vi "Step by Name or ID.vi"(8 "error in (no error)":errorcluster, 10 "Name or ID":string, 11 "Sequence in":refnum<class "Sequence.lvclass">) -> (0 "error out":errorcluster, 2 "Step":refnum<class "Step.lvclass">, 3 "Sequence out":refnum<class "Sequence.lvclass">)   [LabVIEW 2020, in "TSnax.lvlib" / "Sequence.lvclass"]
uses:
  Sequence.lvclass
  Sequence.lvclass/Sequence.ctl
  Step/Step.lvclass
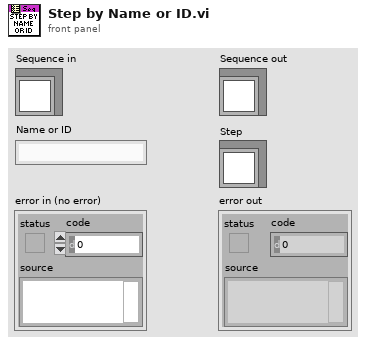
[diagram p1: front panel]
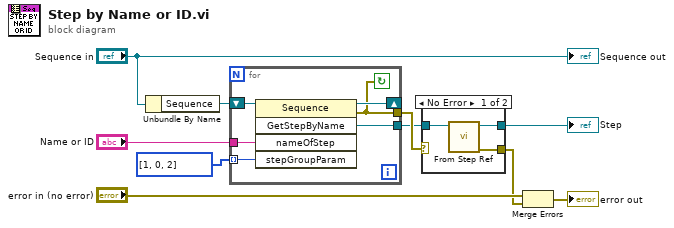
[diagram p0: block diagram]
diagram:
  n1 = Unbundle By Name("Sequence in") -> ("Sequence"=w7:refnum<k7>)
  n2 = for {
    tunnel: "Name or ID" -> [w15]
    tunnel: i32[] [1, 0, 2] -> [w14] mode=indexing
    shift-right: [w13] -> _
    shift-left: w7 -> [w16]
    tunnel: [w12] -> w4
    tunnel: [w11] -> w10
    stop <- w11 continue-if-true
    n3 = invoke class="Sequence" method="GetStepByName"(reference=w16, "nameOfStep"=w15, "stepGroupParam"=w14) -> (reference out=w13:refnum<k7>, error out=w11:errorcluster, "GetStepByName"=w12:refnum<k7>)  [unwired: 2 in, 2 out]
  }
  n4 = case shown="No Error" w10 {
    selector: w10 -> [_ w20]
    tunnel: w4 -> [w19 _]
    tunnel: [w18 w20] -> w1
    tunnel: [w17 _] -> w3
    frame No Error {
      n5 = call "From Step Ref.vi"("Ref"=w19) -> ("error out"=w18:errorcluster, "Step out"=w17:refnum<class "Step.lvclass">)  [unwired: 9 in]
    }
    frame Error {
    }
  }
  "Step" <- w3
  n6 = Merge Errors("error in (no error)", w1) -> (→"error out":errorcluster)
  "Sequence out" <- "Sequence in"
